vi "Transform Outline Points.vi"(8 "error in (no error)":errorcluster, 10 "2xN Matrix":T3, 11 "Outline Glyph Rec":T1) -> (0 "error out":errorcluster, 3 "Outline Glyph Rec dup":T1)   [LabVIEW 2023, in "Freetype Drawer.lvlib"]
uses:
  Freetype Drawer.lvlib
  Outline Glyph Rec.ctl
  Glyph Rec.ctl
  <vilib>/Analysis/Matrix/Datatypes/RealMatrix.ctl
  Get Transformation Components.vi
  Glyph/Glyph Drawer.lvlib
  <vilib>/Analysis/Matrix/NI_Matrix.lvlib
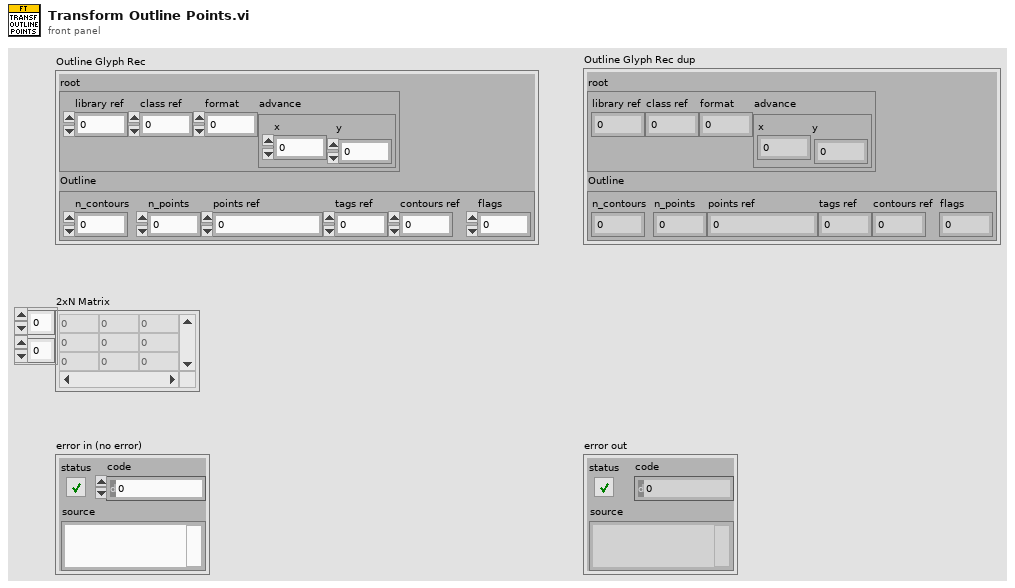
[diagram p1: front panel]
types:
  T1 = typedef "Freetype Drawer.lvlib/Outline Glyph Rec.ctl" = cluster{"root":T2, "Outline":cluster{"n_contours":i16, "n_points":i16, "points ref":i64, "tags ref":i64, "contours ref":i64, "flags":i32}}
  T2 = typedef "Freetype Drawer.lvlib/Glyph Rec.ctl" = cluster{"library ref":i64, "class ref":i64, "format":i32, "advance":cluster{"x":i32, "y":i32}}
  T3 = typedef "NI_Matrix.lvlib/RealMatrix.ctl" = dbl[][]
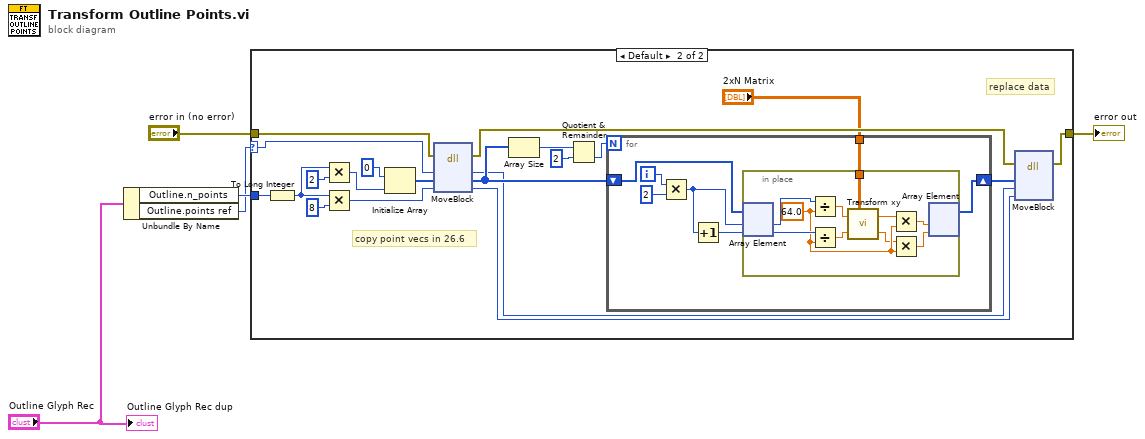
[diagram p0: block diagram]
diagram:
  n1 = Unbundle By Name("Outline Glyph Rec") -> ("Outline.n_points"=w4:i16, "Outline.points ref"=w1:i64)
  n2 = case shown="Default" w1 {
    selector: w1 -> [_ w26]
    tunnel: "error in (no error)" -> [w6 w23]
    tunnel: w4 -> [_ w21]
    tunnel: [w6 w15] -> w3
    frame 0 {
    }
    frame Default {
      # "replace data"
      # "copy point vecs in 26.6"
      n3 = To Long Integer(number=w21) -> (32bit integer=w19:i32)
      n4 = Multiply(x=w19, y=2) -> (x*y=w18:i32)
      n5 = Multiply(x=w19, y=8) -> (x*y=w24:i32)
      n6 = Initialize Array(0 ("x"), w18) -> (w22:i32[])
      n7 = dll-call lib="LabVIEW" fn="MoveBlock"(error in=w23, "src"=w26, "dst"=w22, "size"=w24) -> (error out=w16:errorcluster, "src"=w9:i64, "dst"=w11:i32[], "size"=w8:i32)  [unwired: 3 in, 1 out]
      n8 = Array Size(array=w11) -> (size(s)=w12:i32)
      n9 = Quotient & Remainder(x=w12, y=2) -> (floor(x/y)=w13:i32)  [unwired: 1 out]
      n10 = for {
        N: w13 -> [_]
        shift-right: [w32] -> w10
        shift-left: w11 -> [w33]
        tunnel: "2xN Matrix" -> [w27]
        i -> [w31]
        n11 = Multiply(x=w31, y=2) -> (x*y=w29:i32)
        n12 = Increment(x=w29) -> (x+1=w28:i32)
        n13 = in-place {
          in-place-border: w27 -> [w38]
          w41 = 64.0
          n14 = in-place-array #1(w33, w29, w28) -> (w43:i32, w42:i32)
          n15 = Divide(x=w43, y=w41) -> (x/y=w37:dbl)
          n16 = Divide(x=w42, y=w41) -> (x/y=w36:dbl)
          n17 = call "Transform xy.vi"("y"=w36, "x"=w37, "2xN Matrix"=w38) -> ("y t"=w34:dbl, "x t"=w35:dbl)  [unwired: 1 in]
          n18 = Multiply(x=w35, y=w41) -> (x*y=w40:dbl)
          n19 = Multiply(x=w34, y=w41) -> (x*y=w39:dbl)
          n20 = in-place-array #1(w40, w39) -> (w32:i32[])  [unwired: 2 out]
        }
      }
      n21 = dll-call lib="LabVIEW" fn="MoveBlock"(error in=w16, "src"=w10, "dst"=w9, "size"=w8) -> (error out=w15:errorcluster)  [unwired: 6 in, 1 out]
    }
  }
  "error out" <- w3
  "Outline Glyph Rec dup" <- "Outline Glyph Rec"
